vi "FTW-Time-Display-Timestamp.vi"(3 "Format":T1, 4 "Timestamp (unwired for current time)":timestamp format="%^<%Y-%m-%dT%H:%M:%S%3uZ>T") -> (0 "Formatted Timestamp":string)   [LabVIEW 2015]
uses:
  FTW-Time-DisplayFormat-Timestamp.ctl
panel:
  # "Inputs"
  # "Outputs"
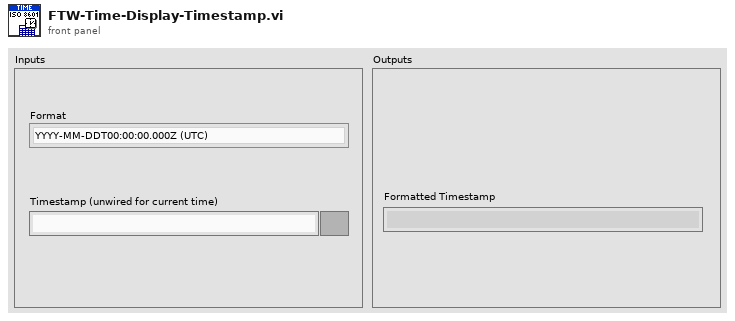
[diagram p1: front panel]
types:
  T1 = typedef "FTW-Time-DisplayFormat-Timestamp.ctl" = enum16{"YYYY-MM-DDT00:00:00.000Z (UTC)", "YYYY-MM-DDT00:00:00.000 (locale)", "YYYY-MM-DDT00:00:00.000+hh:mm (time zone)", "YYYY-MM-DDT00-00-00Z (simple UTC)", "YYYY-MM-DDT00-00-00 (simple locale)", "YYYY-MM-DD"}
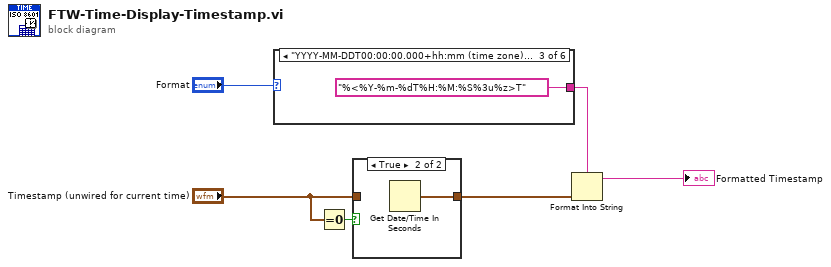
[diagram p0: block diagram]
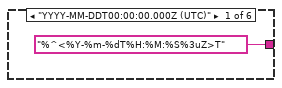
[diagram p2: hidden frame]
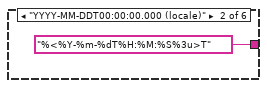
[diagram p3: hidden frame]
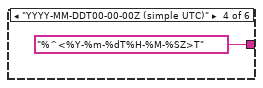
[diagram p4: hidden frame]
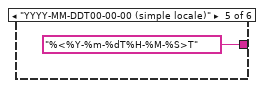
[diagram p5: hidden frame]
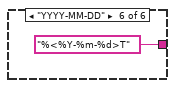
[diagram p6: hidden frame]
diagram:
  n1 = case shown="\"YYYY-MM-DDT00:00:00.000+hh:mm (time zone)\"" "Format" {
    tunnel: ["%^<%Y-%m-%dT%H:%M:%S%3uZ>T" ("format string") "%<%Y-%m-%dT%H:%M:%S%3u>T" ("format string") "%<%Y-%m-%dT%H:%M:%S%3u%z>T" ("format string") "%^<%Y-%m-%dT%H-%M-%SZ>T" ("format string") "%<%Y-%m-%dT%H-%M-%S>T" ("format string") "%<%Y-%m-%d>T" ("format string")] -> w6
    frame "YYYY-MM-DDT00:00:00.000Z (UTC)" {
    }
    frame "YYYY-MM-DDT00:00:00.000 (locale)" {
    }
    frame "YYYY-MM-DDT00:00:00.000+hh:mm (time zone)" {
    }
    frame "YYYY-MM-DDT00-00-00Z (simple UTC)" {
    }
    frame "YYYY-MM-DDT00-00-00 (simple locale)" {
    }
    frame "YYYY-MM-DD" {
    }
  }
  n2 = Equal To 0?(x="Timestamp (unwired for current time)") -> (x = 0?=w4:bool)
  n3 = case shown="True" w4 {
    tunnel: [w13 w14] -> w5
    tunnel: "Timestamp (unwired for current time)" -> [w13 _]
    frame False {
    }
    frame True {
      n4 = Get Date/Time In Seconds() -> (seconds since 1Jan1904=w14:timestamp)
    }
  }
  n5 = Format Into String(format string=w6, w5) -> (resulting string=→"Formatted Timestamp":string)  [unwired: 2 in, 1 out]
